vi "PointMap_DuplicateMap.vi"(8 "error in (no error)":errorcluster, 11 "map in":T1) -> (0 "error out":errorcluster, 3 "duplicate map":T1)   [LabVIEW 2017, in "PointValueMap.lvlib"]
doc: "Copy one maps contents into another map. The destination map is created and will have the exact same contents as the source map."
uses:
  <vilib>/addons/PointValueMap/PointValueMap.lvlib
  <vilib>/addons/PointValueMap/controls/PointMap.ctl
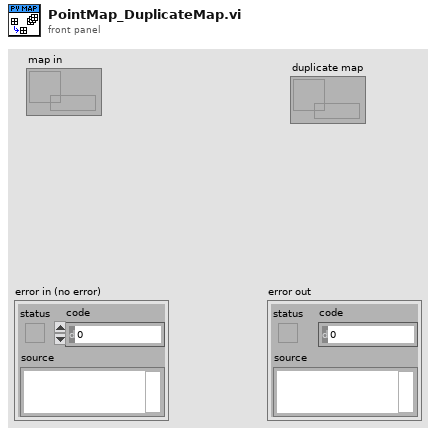
[diagram p1: front panel]
types:
  T1 = typedef "PointValueMap.lvlib/PointMap.ctl" = refnum<data-value>
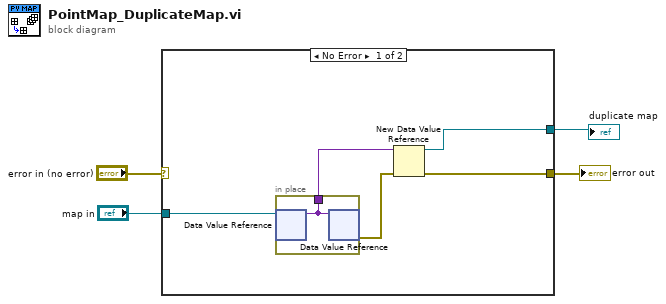
[diagram p0: block diagram]
diagram:
  n1 = case shown="No Error" "error in (no error)" {
    selector: "error in (no error)" -> [_ w11]
    tunnel: [w7 w11] -> w4
    tunnel: [w8 _] -> w2
    tunnel: "map in" -> [w6 _]
    frame No Error {
      n2 = in-place {
        in-place-border: [w10] -> w9
        n3 = in-place-dvr #1(w6) -> (w10:variant)  [unwired: 1 out]
        n4 = in-place-dvr #1(w10) -> (w5:errorcluster)  [unwired: 1 out]
      }
      n5 = New Data Value Reference(data value=w9, error in=w5) -> (data value reference=w8:refnum<data-value>, error out=w7:errorcluster)
    }
    frame Error {
    }
  }
  "error out" <- w4
  "duplicate map" <- w2
